vi "Autonomous Independent.vi"   [LabVIEW 2015]
doc: "This VI is called when autonomous begins, and will automatically be terminated when autonomous ends. You can carry out timed or sensor driven robot movement independently without needing to return to the caller."
uses:
  <vilib>/Rock Robotics/WPI/CAN/TalonSRX/WPI_CANTalonSRX_Params.ctl
  <vilib>/Rock Robotics/Network Tables/NT Read Number.vi
  <vilib>/Rock Robotics/Network Tables/NT Read Boolean.vi
  Robot Global Data.vi
  Team900-VIs/navX Library v2/navX Library v2.lvlib
panel:
  # "Be sure to right-click and choose Data Operations>>Make Current Value default if you want to save the array values with the VI"
types:
  T1 = typedef "WPI_MotorControlDeviceRef.ctl" = cluster{"DeviceStatus":errorcluster, "Type":T2, "PWM":cluster{"PWM Channel":T3, "DeadBand":T4}, "CAN":cluster{"Device Number":u8, "Control Mode":T5, "Semaphore":T6, "Max Vout":dbl, "TalonSRX Control Mode":T7}, "Invert":bool}
  T2 = typedef "WPI_MotorControlType.ctl" = enum16{"PWM", "CAN", "CANTalonSRX"}
  T3 = typedef "FPGA_DIOPWMChannel.ctl" = enum8{"PWM 0", "PWM 1", "PWM 2", "PWM 3", "PWM 4", "PWM 5", "PWM 6", "PWM 7", "PWM 8", "PWM 9", "PWM MXP 0", "PWM MXP 1", "PWM MXP 2", "PWM MXP 3", "PWM MXP 4", "PWM MXP 5", "PWM MXP 6", "PWM MXP 7", "PWM MXP 8", "PWM MXP 9", "Invalid"}
  T4 = typedef "WPI_PWMDeadband.ctl" = cluster{"Name":string, "maxPositivePwm":i32, "minPositivePwm":i32, "centerPwm":i32, "maxNegativePwm":i32, "minNegativePwm":i32, "angularRange":u16}
  T5 = typedef "WPI_CANJaguar_ControlMode.ctl" = enum8{"Percent VBus", "Current", "Speed", "Position", "Voltage"}
  T6 = typedef "Semaphore RefNum" = refnum<k1>
  T7 = typedef "WPI_CANTalonSRX_APIControlMode.ctl" = enum8{"Percent VBus", "Speed", "Position", "Slave", "Unchanged / Invalid", "Voltage Compensation", "Current", "Motion Profile"}
  T8 = typedef "WPI_CANTalonSRX_Params.ctl" = u8
  T9 = typedef "navX Library v2.lvlib/Z900_navX_DeviceTypeDef.ctl" = cluster{"Interface":cluster{"Protocol":T10, "Update Rate (4Hz-60Hz)":u8, "navX Open TypeDef":variant}, "Notify Packet":refnum<notifier>, "Loop VI Refnum":refnum<vi>, "Ready to Close Occurrence Refnum":refnum<k4>}
  T10 = typedef "navX Library v2.lvlib/Z900_navX_ProtocolTypeDef.ctl" = enum16{"SERIAL", "I2C", "SPI"}
  T11 = cluster{"Yaw":dbl, "Roll":dbl, "Pitch":dbl, "Heading":dbl, "Fused Heading":dbl}
  T12 = enum16{"nothing", "Fire", "Aim Goal", "Aim Foward"}
  T13 = enum16{"Nothing", "Turn to Angle", "Pick Up Ball", "Drive Straight", "Drive to Target (arc)"}
  T14 = cluster{"X":dbl, "Y":dbl, "Angle":dbl, "Distance":dbl}
  T15 = enum16{"nothing", "intaketotop", "eject ball", "load ball to shooter", "intaketobottom"}
  T16 = typedef "WPI_DigitalInputDevRef.ctl" = cluster{"DevStatus":errorcluster, "DIO Channel":T17}
  T17 = typedef "FPGA_DIOChannel.ctl" = enum8{"DIO 0", "DIO 1", "DIO 2", "DIO 3", "DIO 4", "DIO 5", "DIO 6", "DIO 7", "DIO 8", "DIO 9", "DIO MXP 0", "DIO MXP 1", "DIO MXP 2", "DIO MXP 3", "DIO MXP 4", "DIO MXP 5", "DIO MXP 6", "DIO MXP 7", "DIO MXP 8", "DIO MXP 9", "DIO MXP 10", "DIO MXP 11", "DIO MXP 12", "DIO MXP 13", "DIO MXP 14", "DIO MXP 15", "Invalid"}
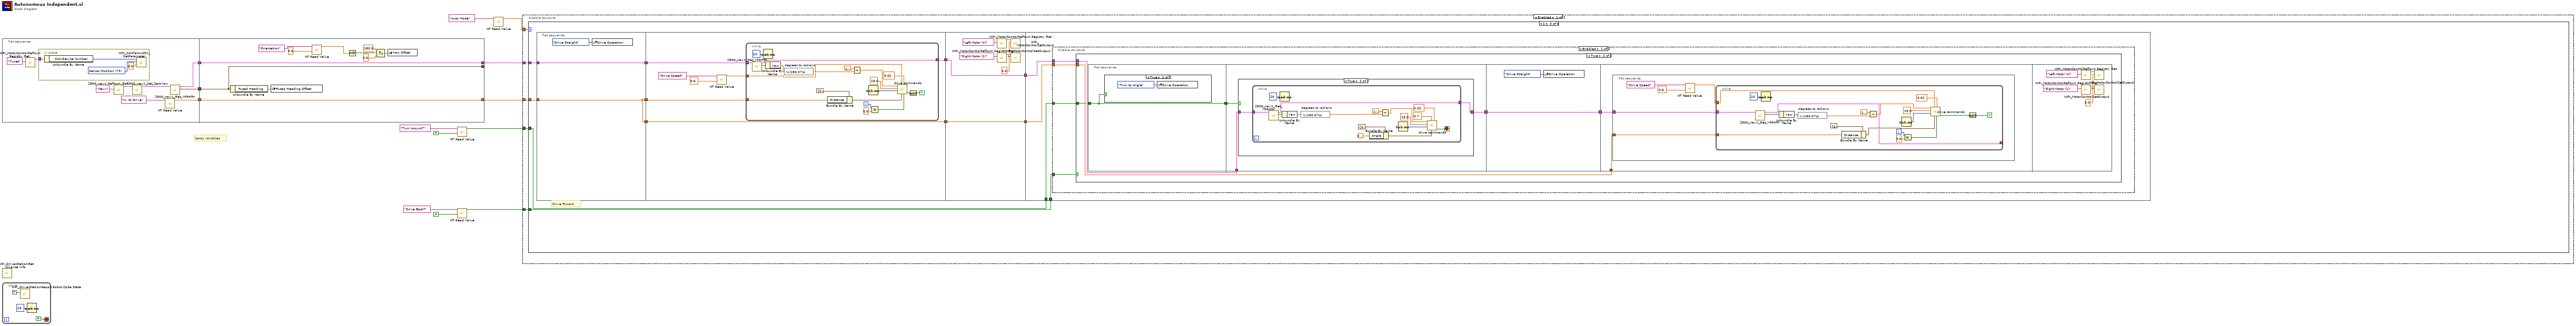
[diagram p0: block diagram]
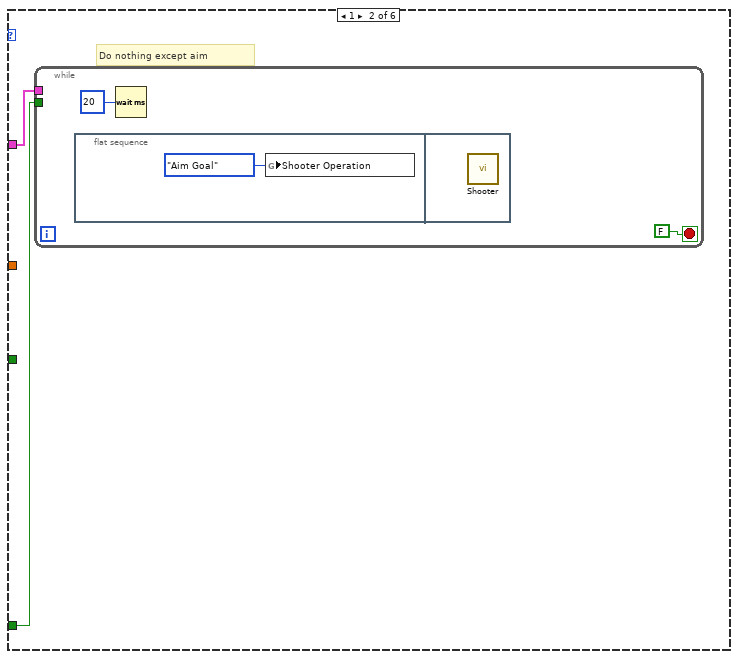
[diagram p3: hidden frame]
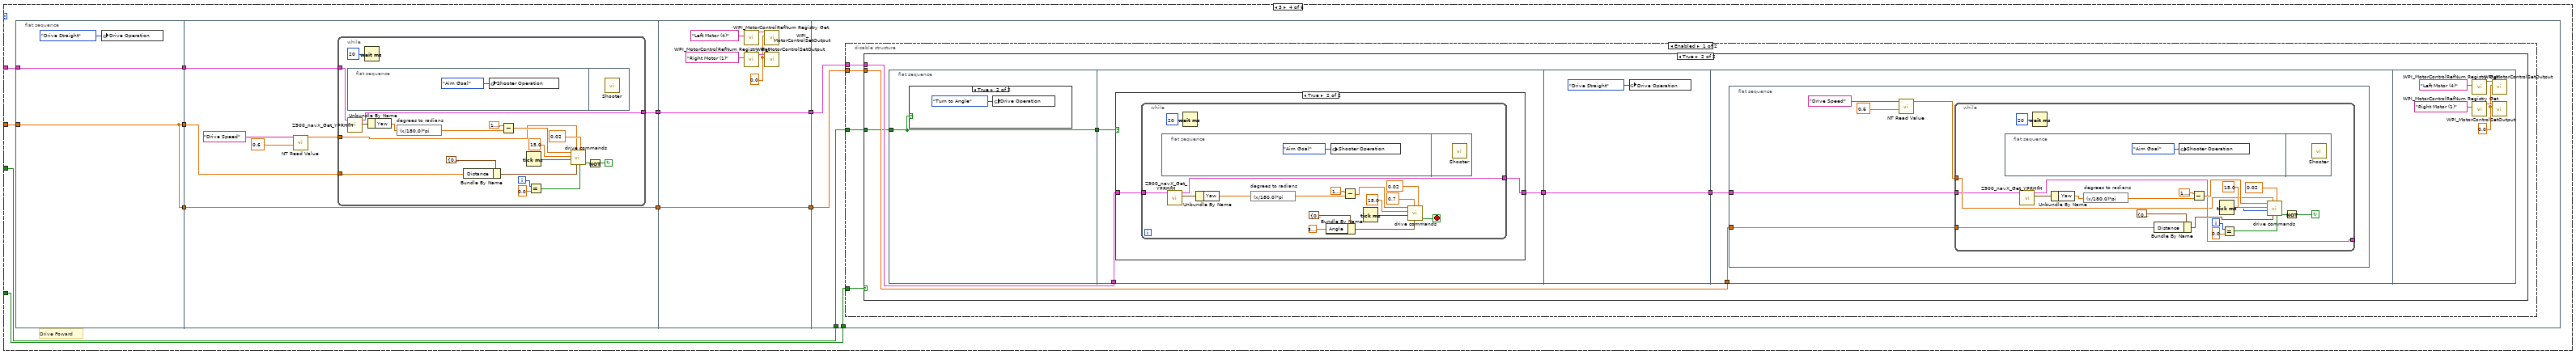
[diagram p8: hidden frame]
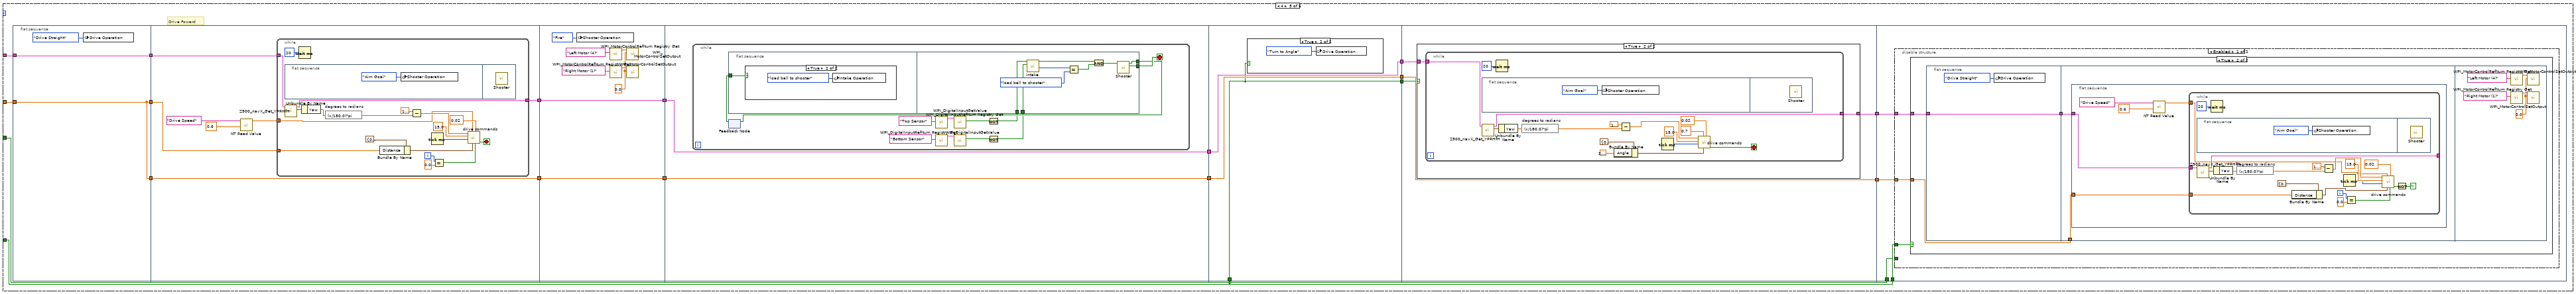
[diagram p13: hidden frame]
diagram:
  # "Zeros variables"
  n1 = flat-sequence {
    tunnel: [w21] -> w3
    tunnel: [w17] -> w2
    tunnel: [w16] -> w1
    tunnel: [w34] -> _
    tunnel: [w36] -> w6
    tunnel: [w37] -> w11
    tunnel: w3 -> [w37]
    tunnel: w2 -> [w36]
    tunnel: w1 -> [w34]
    frame #0 {
      n2 = call <vilib>:"WPI_MotorControlRefNum Registry Get.vi"("refnum name"="Turret") -> ("MotorControlDevRef"=w15:T1)  [unwired: 9 in, 1 out]
      n3 = in-place {
        in-place-border: w15 -> [w26]
        w24 = T8 73 items=["Slot 0 - P"=1, "Slot 0 - I"=2, "Slot 0 - D"=3, "Slot 0 - F"=4, "Slot 0 - I Zone"=5, "Slot 0 - Ramp Rate"=6, "Slot 1 - P"=11, "Slot 1 - I"=12, "Slot 1 - D"=13, "Slot 1 - F"=14, "Slot 1 - I Zone"=15, "Slot 1 - Ramp Rate"=16, "Soft Limit - Forward"=21, "Soft Limit - Reverse"=22, "On Boot - Brake Mode"=31, "On Boot - Limit Normally Closed - Forward"=32, "On Boot - Limit Normally Closed - Reverse"=33, "On Boot - Limit Disabled - Forward"=34, "On Boot - Limit Disabled - Reverse"=35, "Fault - Over Temp"=41, "Fault - Under Voltage"=42, "Fault - Forward Limit"=43, "Fault - Reverse Limit"=44, "Fault - Hardware Failure"=45, "Fault - Forward Soft Limit"=46, "Fault - Reverse Soft Limit"=47, "Sticky Fault - Over Temp"=48, "Sticky Fault - Under Voltage"=49, "Sticky Fault - Forward Limit"=50, "Sticky Fault - Reverse Limit"=51, "Sticky Fault - Forward Soft Limit"=52, "Sticky Fault - Reverse Soft Limit"=53, "Applied Throttle"=61, "Closed-Loop Error"=62, "Select Feedback Device"=63, "Reverse Closed-Loop Output"=64, "Mode Select"=65, "Profile Slot Select"=66, "Ramp Throttle"=67, "Reverse Feedback Sensor"=68, "Limit Switch Enabled"=69, "Limit Switch Closed - Forward"=70, "Limit Switch Closed - Reverse"=71, "Sensor Position"=73, "Sensor Velocity"=74, "Current"=75, "Brake is Enabled"=76, "Encoder Position"=77, "Encoder Velocity"=78, "Encoder Index Rise Events"=79, "Encoder A Pin State"=80, "Encoder B Pin State"=81, "Encoder Index Pin State"=82, "Analog In with Overflow"=83, "Analog In Velocity"=84, "Temperature"=85, "Battery Voltage"=86, "Reset Count"=87, "Reset Flags"=88, "Firmware Version"=89, "Settings Changed"=90] ("Parameter")
        n4 = Unbundle By Name(w26) -> ("CAN.Device Number"=w25:u8)
        n5 = call <vilib>:"WPI_CANTalonSRX_SetParameter.vi"("Value"=0.0, "Parameter"=w24, "Device ID (0)"=w25) -> ()  [unwired: 7 in, 2 out]
      }
      n6 = call "Z900_navX_RefNum_Get.vi"("refnum name"="Navx") -> ("navX Device"=w19:T9)  [unwired: 9 in, 1 out]
      n7 = call "Z900_navX_Set_ZeroYaw.vi"("navX Device"=w19) -> ("navX Device"=w18:T9)  [unwired: 9 in, 1 out]
      n8 = call-poly <vilib>:"NT Read Value.vi"("Name"="In. to Drive") -> ("Numeric"=w21:dbl)  [unwired: 9 in, 1 out]
      n9 = call "Z900_navX_Get_YPRHfH.vi"("navX Device"=w18) -> ("YRPHfH"=w16:T11, "navX Device"=w17:T9)  [unwired: 7 in, 2 out]
    }
    frame #1 {
      n10 = Unbundle By Name(w34) -> ("Fused Heading"=w35:dbl)
      n11 = global write "Robot Global Data.vi" "Fused Heading Offset"(w35) -> ()
      n12 = call-poly <vilib>:"NT Read Value.vi"("Default Value"=0.0, "Name"="Orientation") -> ("Numeric"=w32:dbl)  [unwired: 8 in, 1 out]
      n13 = Equal To 0?(x=w32) -> (x = 0?=w31:bool)
      n14 = Select(t=180.0, s=w31, f=0.0) -> (s? t:f=w28:dbl)
      n15 = global write "Robot Global Data.vi" "Yaw Offset"(w28) -> ()
    }
  }
  n16 = call <vilib>:"WPI_DriverStationGet Alliance Info.vi"() -> ()  [unwired: 12 out]
  n17 = while {
    stop <- FALSE stop-if-true
    n18 = call <vilib>:"WPI_DriverStationReport Robot Code State.vi"("Autonomous"=TRUE) -> ()  [unwired: 10 in, 1 out]
    n19 = Wait (ms)(milliseconds to wait=u32 20) -> ()  [unwired: 1 out]
  }
  n20 = call-poly <vilib>:"NT Read Value.vi"("Default Value"=FALSE, "Name"="Turn Around?") -> ("Boolean"=w7:bool)  [unwired: 8 in, 1 out]
  n21 = call-poly <vilib>:"NT Read Value.vi"("Default Value"=FALSE, "Name"="Drive Back?") -> ("Boolean"=w10:bool)  [unwired: 8 in, 1 out]
  n22 = call-poly <vilib>:"NT Read Value.vi"("Name"="Auto Mode") -> ("Numeric"=w5:dbl)  [unwired: 9 in, 1 out]
  n23 = disable-structure shown="Enabled" {
    disable-tunnel: w5 -> [w45 _]
    disable-tunnel: w6 -> [w44 _]
    disable-tunnel: w11 -> [w43 _]
    disable-tunnel: w10 -> [w42 _]
    disable-tunnel: w7 -> [w41 _]
    frame Enabled {
      n24 = case shown="2" w45 {
        tunnel: w44 -> [_ w47 w61 w181 w311 _]
        tunnel: w43 -> [_ _ w60 w180 w310 _]
        tunnel: w42 -> [_ w46 w57 w177 w307 _]
        tunnel: w41 -> [_ _ w51 w171 w295 _]
        frame 0, Default {
          # "Do nothing"
        }
        frame 1 {
          # "Do nothing except aim"
          n25 = while {
            tunnel: w47 -> [_]
            tunnel: w46 -> [_]
            stop <- FALSE stop-if-true
            n26 = flat-sequence {
              frame #0 {
                n27 = global write "Robot Global Data.vi" "Shooter Operation"(T12."Aim Goal" ("Shooter Operation")) -> ()
              }
              frame #1 {
                n28 = call "Shooter.vi"() -> ()  [unwired: 8 in, 4 out]
              }
            }
            n29 = Wait (ms)(milliseconds to wait=20) -> ()  [unwired: 1 out]
          }
        }
        frame 2 {
          # "Drive Foward"
          n30 = flat-sequence {
            tunnel: w60 -> [w62]
            tunnel: w61 -> [w64]
            tunnel: [w64] -> w59
            tunnel: [w62] -> w58
            tunnel: [w62] -> w54
            tunnel: w59 -> [w71]
            tunnel: w58 -> [w70]
            tunnel: [w69] -> w56
            tunnel: w54 -> [w65]
            tunnel: [w65] -> w53
            tunnel: w56 -> [w98]
            tunnel: [w98] -> w55
            tunnel: w53 -> [w92]
            tunnel: [w92] -> w52
            tunnel: w57 -> [w102]
            tunnel: w55 -> [w101]
            tunnel: w52 -> [w100]
            tunnel: w51 -> [w99]
            frame #0 {
              n31 = global write "Robot Global Data.vi" "Drive Operation"(T13."Drive Straight" ("Drive Operation")) -> ()
            }
            frame #1 {
              n32 = call-poly <vilib>:"NT Read Value.vi"("Default Value"=0.6, "Name"="Drive Speed") -> ("Numeric"=w66:dbl)  [unwired: 8 in, 1 out]
              n33 = while {
                tunnel: w71 -> [w91]
                tunnel: w70 -> [w83]
                tunnel: [w78] -> w69
                tunnel: w66 -> [w72]
                i -> [w75]
                stop <- w76 continue-if-true
                n34 = call "Z900_navX_Get_YPRHfH.vi"("navX Device"=w91) -> ("YRPHfH"=w90:T11, "navX Device"=w78:T9)  [unwired: 7 in, 2 out]
                n35 = Wait (ms)(milliseconds to wait=20) -> ()  [unwired: 1 out]
                n36 = Unbundle By Name(w90) -> ("Yaw"=w87:dbl)
                n37 = expression code="(x/180.0)*pi" "degrees to radians"(w87) -> (w86:dbl)
                n38 = Bundle By Name(cluster=T14 {"X"=0.0, "Y"=0.0, "Angle"=0.0, "Distance"=0.0} ("Position"), "Distance"=w83) -> (w81:T14)
                n39 = Subtract(x=1.5707963267948966, y=w86) -> (x-y=w89:dbl)
                n40 = Tick Count (ms)() -> (millisecond timer value=w84:u32)
                n41 = Equal?(x=w75, y=0.0) -> (x = y?=w73:bool)
                n42 = call "drive commands.vi"("New Command"=w73, "Angle Tolerance"=0.02, "Position"=w81, "Speed Setpoint"=w72, "Current Time"=w84, "Duration"=15.0, "Yaw (radians, 0=right)"=w89) -> ("Finished"=w79:bool)  [unwired: 2 in, 2 out]
                n43 = Not(x=w79) -> (.not. x?=w76:bool)
              }
            }
            frame #2 {
              w93 = 0.0 ("Output")
              n44 = call <vilib>:"WPI_MotorControlRefNum Registry Get.vi"("refnum name"="Left Motor (4)") -> ("MotorControlDevRef"=w94:T1)  [unwired: 9 in, 1 out]
              n45 = call <vilib>:"WPI_MotorControlRefNum Registry Get.vi"("refnum name"="Right Motor (1)") -> ("MotorControlDevRef"=w95:T1)  [unwired: 9 in, 1 out]
              n46 = call <vilib>:"WPI_MotorControlSetOutput.vi"("Output"=w93, "MotorControlDevRef"=w94) -> ()  [unwired: 7 in, 3 out]
              n47 = call <vilib>:"WPI_MotorControlSetOutput.vi"("Output"=w93, "MotorControlDevRef"=w95) -> ()  [unwired: 7 in, 3 out]
            }
            frame #3 {
              n48 = disable-structure shown="Enabled" {
                disable-tunnel: w102 -> [w106 _]
                disable-tunnel: w101 -> [w105 _]
                disable-tunnel: w100 -> [w104 _]
                disable-tunnel: w99 -> [w103 _]
                frame Enabled {
                  n49 = case shown="True" w106 {
                    tunnel: w105 -> [_ w112]
                    tunnel: w104 -> [_ w110]
                    tunnel: w103 -> [_ w109]
                    frame False {
                    }
                    frame True {
                      n50 = flat-sequence {
                        tunnel: w109 -> [w113]
                        tunnel: [w113] -> w108
                        tunnel: w112 -> [w117]
                        tunnel: [w116] -> w111
                        tunnel: w108 -> [w115]
                        tunnel: w111 -> [w137]
                        tunnel: [w137] -> w107
                        tunnel: w110 -> [w140]
                        tunnel: w107 -> [w139]
                        frame #0 {
                          n51 = case shown="True" w113 {
                            frame False {
                            }
                            frame True {
                              n52 = global write "Robot Global Data.vi" "Drive Operation"(T13."Turn to Angle" ("Drive Operation")) -> ()
                            }
                          }
                        }
                        frame #1 {
                          n53 = case shown="True" w115 {
                            tunnel: w117 -> [w118 w120]
                            tunnel: [w118 w119] -> w116
                            frame False {
                            }
                            frame True {
                              n54 = while {
                                tunnel: w120 -> [w136]
                                tunnel: [w121] -> w119
                                stop <- w124 stop-if-true
                                n55 = call "Z900_navX_Get_YPRHfH.vi"("navX Device"=w136) -> ("YRPHfH"=w135:T11, "navX Device"=w121:T9)  [unwired: 7 in, 2 out]
                                n56 = Wait (ms)(milliseconds to wait=20) -> ()  [unwired: 1 out]
                                n57 = Unbundle By Name(w135) -> ("Yaw"=w132:dbl)
                                n58 = expression code="(x/180.0)*pi" "degrees to radians"(w132) -> (w131:dbl)
                                n59 = Bundle By Name(cluster=T14 {"X"=0.0, "Y"=0.0, "Angle"=0.0, "Distance"=0.0} ("Position"), "Angle"=3.141592653589793) -> (w127:T14)
                                n60 = Subtract(x=1.5707963267948966, y=w131) -> (x-y=w134:dbl)
                                n61 = Tick Count (ms)() -> (millisecond timer value=w129:u32)
                                n62 = call "drive commands.vi"("Angle Tolerance"=0.02, "Position"=w127, "Speed Setpoint"=0.7, "Current Time"=w129, "Duration"=15.0, "Yaw (radians, 0=right)"=w134) -> ("Finished"=w124:bool)  [unwired: 3 in, 2 out]
                              }
                            }
                          }
                        }
                        frame #2 {
                          n63 = global write "Robot Global Data.vi" "Drive Operation"(T13."Drive Straight" ("Drive Operation")) -> ()
                        }
                        frame #3 {
                          n64 = flat-sequence {
                            tunnel: w140 -> [w142]
                            tunnel: w139 -> [w141]
                            frame #0 {
                              n65 = call-poly <vilib>:"NT Read Value.vi"("Default Value"=0.6, "Name"="Drive Speed") -> ("Numeric"=w143:dbl)  [unwired: 8 in, 1 out]
                              n66 = while {
                                tunnel: [w154] -> _
                                tunnel: w143 -> [w148]
                                tunnel: w142 -> [w147]
                                tunnel: w141 -> [w146]
                                i -> [w151]
                                stop <- w152 continue-if-true
                                n67 = call "Z900_navX_Get_YPRHfH.vi"("navX Device"=w146) -> ("YRPHfH"=w165:T11, "navX Device"=w154:T9)  [unwired: 7 in, 2 out]
                                n68 = Wait (ms)(milliseconds to wait=20) -> ()  [unwired: 1 out]
                                n69 = Unbundle By Name(w165) -> ("Yaw"=w162:dbl)
                                n70 = expression code="(x/180.0)*pi" "degrees to radians"(w162) -> (w161:dbl)
                                n71 = Bundle By Name(cluster=T14 {"X"=0.0, "Y"=0.0, "Angle"=0.0, "Distance"=0.0} ("Position"), "Distance"=w147) -> (w157:T14)
                                n72 = Subtract(x=1.5707963267948966, y=w161) -> (x-y=w164:dbl)
                                n73 = Tick Count (ms)() -> (millisecond timer value=w159:u32)
                                n74 = Equal?(x=w151, y=0.0) -> (x = y?=w149:bool)
                                n75 = call "drive commands.vi"("New Command"=w149, "Angle Tolerance"=0.02, "Position"=w157, "Speed Setpoint"=w148, "Current Time"=w159, "Duration"=15.0, "Yaw (radians, 0=right)"=w164) -> ("Finished"=w155:bool)  [unwired: 2 in, 2 out]
                                n76 = Not(x=w155) -> (.not. x?=w152:bool)
                              }
                            }
                          }
                        }
                        frame #4 {
                          w166 = 0.0 ("Output")
                          n77 = call <vilib>:"WPI_MotorControlRefNum Registry Get.vi"("refnum name"="Left Motor (4)") -> ("MotorControlDevRef"=w167:T1)  [unwired: 9 in, 1 out]
                          n78 = call <vilib>:"WPI_MotorControlRefNum Registry Get.vi"("refnum name"="Right Motor (1)") -> ("MotorControlDevRef"=w168:T1)  [unwired: 9 in, 1 out]
                          n79 = call <vilib>:"WPI_MotorControlSetOutput.vi"("Output"=w166, "MotorControlDevRef"=w167) -> ()  [unwired: 7 in, 3 out]
                          n80 = call <vilib>:"WPI_MotorControlSetOutput.vi"("Output"=w166, "MotorControlDevRef"=w168) -> ()  [unwired: 7 in, 3 out]
                        }
                      }
                    }
                  }
                }
                frame Disabled {
                }
              }
            }
          }
        }
        frame 3 {
          # "Drive Foward"
          n81 = flat-sequence {
            tunnel: w180 -> [w182]
            tunnel: w181 -> [w184]
            tunnel: [w184] -> w179
            tunnel: [w182] -> w178
            tunnel: [w182] -> w174
            tunnel: w179 -> [w191]
            tunnel: w178 -> [w190]
            tunnel: [w189] -> w176
            tunnel: w174 -> [w185]
            tunnel: [w185] -> w173
            tunnel: w176 -> [w219]
            tunnel: [w219] -> w175
            tunnel: w173 -> [w213]
            tunnel: [w213] -> w172
            tunnel: w177 -> [w223]
            tunnel: w175 -> [w222]
            tunnel: w172 -> [w221]
            tunnel: w171 -> [w220]
            frame #0 {
              n82 = global write "Robot Global Data.vi" "Drive Operation"(T13."Drive Straight" ("Drive Operation")) -> ()
            }
            frame #1 {
              n83 = call-poly <vilib>:"NT Read Value.vi"("Default Value"=0.6, "Name"="Drive Speed") -> ("Numeric"=w186:dbl)  [unwired: 8 in, 1 out]
              n84 = while {
                tunnel: w191 -> [w211]
                tunnel: w190 -> [w203]
                tunnel: [w198] -> w189
                tunnel: w186 -> [w192]
                i -> [w195]
                stop <- w196 continue-if-true
                n85 = flat-sequence {
                  frame #0 {
                    n86 = global write "Robot Global Data.vi" "Shooter Operation"(T12."Aim Goal" ("Shooter Operation")) -> ()
                  }
                  frame #1 {
                    n87 = call "Shooter.vi"() -> ()  [unwired: 8 in, 4 out]
                  }
                }
                n88 = call "Z900_navX_Get_YPRHfH.vi"("navX Device"=w211) -> ("YRPHfH"=w210:T11, "navX Device"=w198:T9)  [unwired: 7 in, 2 out]
                n89 = Wait (ms)(milliseconds to wait=20) -> ()  [unwired: 1 out]
                n90 = Unbundle By Name(w210) -> ("Yaw"=w207:dbl)
                n91 = expression code="(x/180.0)*pi" "degrees to radians"(w207) -> (w206:dbl)
                n92 = Bundle By Name(cluster=T14 {"X"=0.0, "Y"=0.0, "Angle"=0.0, "Distance"=0.0} ("Position"), "Distance"=w203) -> (w201:T14)
                n93 = Subtract(x=1.5707963267948966, y=w206) -> (x-y=w209:dbl)
                n94 = Tick Count (ms)() -> (millisecond timer value=w204:u32)
                n95 = Equal?(x=w195, y=0.0) -> (x = y?=w193:bool)
                n96 = call "drive commands.vi"("New Command"=w193, "Angle Tolerance"=0.02, "Position"=w201, "Speed Setpoint"=w192, "Current Time"=w204, "Duration"=15.0, "Yaw (radians, 0=right)"=w209) -> ("Finished"=w199:bool)  [unwired: 2 in, 2 out]
                n97 = Not(x=w199) -> (.not. x?=w196:bool)
              }
            }
            frame #2 {
              w214 = 0.0 ("Output")
              n98 = call <vilib>:"WPI_MotorControlRefNum Registry Get.vi"("refnum name"="Left Motor (4)") -> ("MotorControlDevRef"=w215:T1)  [unwired: 9 in, 1 out]
              n99 = call <vilib>:"WPI_MotorControlRefNum Registry Get.vi"("refnum name"="Right Motor (1)") -> ("MotorControlDevRef"=w216:T1)  [unwired: 9 in, 1 out]
              n100 = call <vilib>:"WPI_MotorControlSetOutput.vi"("Output"=w214, "MotorControlDevRef"=w215) -> ()  [unwired: 7 in, 3 out]
              n101 = call <vilib>:"WPI_MotorControlSetOutput.vi"("Output"=w214, "MotorControlDevRef"=w216) -> ()  [unwired: 7 in, 3 out]
            }
            frame #3 {
              n102 = disable-structure shown="Enabled" {
                disable-tunnel: w223 -> [w227 _]
                disable-tunnel: w222 -> [w226 _]
                disable-tunnel: w221 -> [w225 _]
                disable-tunnel: w220 -> [w224 _]
                frame Enabled {
                  n103 = case shown="True" w227 {
                    tunnel: w226 -> [_ w233]
                    tunnel: w225 -> [_ w231]
                    tunnel: w224 -> [_ w230]
                    frame False {
                    }
                    frame True {
                      n104 = flat-sequence {
                        tunnel: w230 -> [w234]
                        tunnel: [w234] -> w229
                        tunnel: w233 -> [w238]
                        tunnel: [w237] -> w232
                        tunnel: w229 -> [w236]
                        tunnel: w232 -> [w259]
                        tunnel: [w259] -> w228
                        tunnel: w231 -> [w262]
                        tunnel: w228 -> [w261]
                        frame #0 {
                          n105 = case shown="True" w234 {
                            frame False {
                            }
                            frame True {
                              n106 = global write "Robot Global Data.vi" "Drive Operation"(T13."Turn to Angle" ("Drive Operation")) -> ()
                            }
                          }
                        }
                        frame #1 {
                          n107 = case shown="True" w236 {
                            tunnel: w238 -> [w239 w241]
                            tunnel: [w239 w240] -> w237
                            frame False {
                            }
                            frame True {
                              n108 = while {
                                tunnel: w241 -> [w257]
                                tunnel: [w242] -> w240
                                stop <- w245 stop-if-true
                                n109 = flat-sequence {
                                frame #0 {
                                n110 = global write "Robot Global Data.vi" "Shooter Operation"(T12."Aim Goal" ("Shooter Operation")) -> ()
                                }
                                frame #1 {
                                n111 = call "Shooter.vi"() -> ()  [unwired: 8 in, 4 out]
                                }
                                }
                                n112 = call "Z900_navX_Get_YPRHfH.vi"("navX Device"=w257) -> ("YRPHfH"=w256:T11, "navX Device"=w242:T9)  [unwired: 7 in, 2 out]
                                n113 = Wait (ms)(milliseconds to wait=20) -> ()  [unwired: 1 out]
                                n114 = Unbundle By Name(w256) -> ("Yaw"=w253:dbl)
                                n115 = expression code="(x/180.0)*pi" "degrees to radians"(w253) -> (w252:dbl)
                                n116 = Bundle By Name(cluster=T14 {"X"=0.0, "Y"=0.0, "Angle"=0.0, "Distance"=0.0} ("Position"), "Angle"=3.141592653589793) -> (w248:T14)
                                n117 = Subtract(x=1.5707963267948966, y=w252) -> (x-y=w255:dbl)
                                n118 = Tick Count (ms)() -> (millisecond timer value=w250:u32)
                                n119 = call "drive commands.vi"("Angle Tolerance"=0.02, "Position"=w248, "Speed Setpoint"=0.7, "Current Time"=w250, "Duration"=15.0, "Yaw (radians, 0=right)"=w255) -> ("Finished"=w245:bool)  [unwired: 3 in, 2 out]
                              }
                            }
                          }
                        }
                        frame #2 {
                          n120 = global write "Robot Global Data.vi" "Drive Operation"(T13."Drive Straight" ("Drive Operation")) -> ()
                        }
                        frame #3 {
                          n121 = flat-sequence {
                            tunnel: w262 -> [w264]
                            tunnel: w261 -> [w263]
                            frame #0 {
                              n122 = call-poly <vilib>:"NT Read Value.vi"("Default Value"=0.6, "Name"="Drive Speed") -> ("Numeric"=w265:dbl)  [unwired: 8 in, 1 out]
                              n123 = while {
                                tunnel: [w276] -> _
                                tunnel: w265 -> [w270]
                                tunnel: w264 -> [w269]
                                tunnel: w263 -> [w268]
                                i -> [w273]
                                stop <- w274 continue-if-true
                                n124 = flat-sequence {
                                frame #0 {
                                n125 = global write "Robot Global Data.vi" "Shooter Operation"(T12."Aim Goal" ("Shooter Operation")) -> ()
                                }
                                frame #1 {
                                n126 = call "Shooter.vi"() -> ()  [unwired: 8 in, 4 out]
                                }
                                }
                                n127 = call "Z900_navX_Get_YPRHfH.vi"("navX Device"=w268) -> ("YRPHfH"=w287:T11, "navX Device"=w276:T9)  [unwired: 7 in, 2 out]
                                n128 = Wait (ms)(milliseconds to wait=20) -> ()  [unwired: 1 out]
                                n129 = Unbundle By Name(w287) -> ("Yaw"=w284:dbl)
                                n130 = expression code="(x/180.0)*pi" "degrees to radians"(w284) -> (w283:dbl)
                                n131 = Bundle By Name(cluster=T14 {"X"=0.0, "Y"=0.0, "Angle"=0.0, "Distance"=0.0} ("Position"), "Distance"=w269) -> (w279:T14)
                                n132 = Subtract(x=1.5707963267948966, y=w283) -> (x-y=w286:dbl)
                                n133 = Tick Count (ms)() -> (millisecond timer value=w281:u32)
                                n134 = Equal?(x=w273, y=0.0) -> (x = y?=w271:bool)
                                n135 = call "drive commands.vi"("New Command"=w271, "Angle Tolerance"=0.02, "Position"=w279, "Speed Setpoint"=w270, "Current Time"=w281, "Duration"=15.0, "Yaw (radians, 0=right)"=w286) -> ("Finished"=w277:bool)  [unwired: 2 in, 2 out]
                                n136 = Not(x=w277) -> (.not. x?=w274:bool)
                              }
                            }
                          }
                        }
                        frame #4 {
                          w289 = 0.0 ("Output")
                          n137 = call <vilib>:"WPI_MotorControlRefNum Registry Get.vi"("refnum name"="Left Motor (4)") -> ("MotorControlDevRef"=w290:T1)  [unwired: 9 in, 1 out]
                          n138 = call <vilib>:"WPI_MotorControlRefNum Registry Get.vi"("refnum name"="Right Motor (1)") -> ("MotorControlDevRef"=w291:T1)  [unwired: 9 in, 1 out]
                          n139 = call <vilib>:"WPI_MotorControlSetOutput.vi"("Output"=w289, "MotorControlDevRef"=w290) -> ()  [unwired: 7 in, 3 out]
                          n140 = call <vilib>:"WPI_MotorControlSetOutput.vi"("Output"=w289, "MotorControlDevRef"=w291) -> ()  [unwired: 7 in, 3 out]
                        }
                      }
                    }
                  }
                }
                frame Disabled {
                }
              }
            }
          }
        }
        frame 4 {
          # "Drive Foward"
          n141 = flat-sequence {
            tunnel: w310 -> [w312]
            tunnel: w311 -> [w314]
            tunnel: [w314] -> w309
            tunnel: [w312] -> w308
            tunnel: [w312] -> w305
            tunnel: w309 -> [w321]
            tunnel: w308 -> [w320]
            tunnel: [w319] -> w306
            tunnel: w305 -> [w315]
            tunnel: [w315] -> w304
            tunnel: w306 -> [w349]
            tunnel: [w349] -> w303
            tunnel: w304 -> [w343]
            tunnel: [w343] -> w302
            tunnel: w303 -> [w351]
            tunnel: [w351] -> w301
            tunnel: w302 -> [w350]
            tunnel: [w350] -> w300
            tunnel: w301 -> [w376]
            tunnel: [w376] -> w299
            tunnel: w300 -> [w375]
            tunnel: [w375] -> w297
            tunnel: w295 -> [w374]
            tunnel: [w374] -> w294
            tunnel: w299 -> [w380]
            tunnel: [w379] -> w298
            tunnel: w297 -> [w381]
            tunnel: [w381] -> w296
            tunnel: w294 -> [w378]
            tunnel: w307 -> [w405]
            tunnel: w298 -> [w404]
            tunnel: w296 -> [w403]
            tunnel: w295 -> [w402]
            frame #0 {
              n142 = global write "Robot Global Data.vi" "Drive Operation"(T13."Drive Straight" ("Drive Operation")) -> ()
            }
            frame #1 {
              n143 = call-poly <vilib>:"NT Read Value.vi"("Default Value"=0.6, "Name"="Drive Speed") -> ("Numeric"=w316:dbl)  [unwired: 8 in, 1 out]
              n144 = while {
                tunnel: w321 -> [w340]
                tunnel: w320 -> [w332]
                tunnel: [w328] -> w319
                tunnel: w316 -> [w323]
                i -> [w326]
                stop <- w322 stop-if-true
                n145 = flat-sequence {
                  frame #0 {
                    n146 = global write "Robot Global Data.vi" "Shooter Operation"(T12."Aim Goal" ("Shooter Operation")) -> ()
                  }
                  frame #1 {
                    n147 = call "Shooter.vi"() -> ()  [unwired: 8 in, 4 out]
                  }
                }
                n148 = call "Z900_navX_Get_YPRHfH.vi"("navX Device"=w340) -> ("YRPHfH"=w339:T11, "navX Device"=w328:T9)  [unwired: 7 in, 2 out]
                n149 = Wait (ms)(milliseconds to wait=20) -> ()  [unwired: 1 out]
                n150 = Unbundle By Name(w339) -> ("Yaw"=w336:dbl)
                n151 = expression code="(x/180.0)*pi" "degrees to radians"(w336) -> (w335:dbl)
                n152 = Bundle By Name(cluster=T14 {"X"=0.0, "Y"=0.0, "Angle"=0.0, "Distance"=0.0} ("Position"), "Distance"=w332) -> (w330:T14)
                n153 = Subtract(x=1.5707963267948966, y=w335) -> (x-y=w338:dbl)
                n154 = Tick Count (ms)() -> (millisecond timer value=w333:u32)
                n155 = Equal?(x=w326, y=0.0) -> (x = y?=w324:bool)
                n156 = call "drive commands.vi"("New Command"=w324, "Angle Tolerance"=0.02, "Position"=w330, "Speed Setpoint"=w323, "Current Time"=w333, "Duration"=15.0, "Yaw (radians, 0=right)"=w338) -> ("Finished"=w322:bool)  [unwired: 2 in, 2 out]
              }
            }
            frame #2 {
              w344 = 0.0 ("Output")
              n157 = global write "Robot Global Data.vi" "Shooter Operation"(T12."Fire" ("Shooter Operation")) -> ()
              n158 = call <vilib>:"WPI_MotorControlRefNum Registry Get.vi"("refnum name"="Left Motor (4)") -> ("MotorControlDevRef"=w345:T1)  [unwired: 9 in, 1 out]
              n159 = call <vilib>:"WPI_MotorControlRefNum Registry Get.vi"("refnum name"="Right Motor (1)") -> ("MotorControlDevRef"=w346:T1)  [unwired: 9 in, 1 out]
              n160 = call <vilib>:"WPI_MotorControlSetOutput.vi"("Output"=w344, "MotorControlDevRef"=w345) -> ()  [unwired: 7 in, 3 out]
              n161 = call <vilib>:"WPI_MotorControlSetOutput.vi"("Output"=w344, "MotorControlDevRef"=w346) -> ()  [unwired: 7 in, 3 out]
            }
            frame #3 {
              n162 = while {
                stop <- w362 stop-if-true
                n163 = flat-sequence {
                  tunnel: w360 -> [w363]
                  tunnel: [w373] -> w362
                  tunnel: [w367] -> w361
                  tunnel: w353 -> [w366]
                  tunnel: w352 -> [w365]
                  frame #0 {
                    n164 = case shown="True" w363 {
                      frame False {
                      }
                      frame True {
                        n165 = global write "Robot Global Data.vi" "Intake Operation"(T15."load ball to shooter" ("Intake Operation")) -> ()
                      }
                    }
                  }
                  frame #1 {
                    n166 = call "intake.vi"("Bottom Sensor"=w365, "Top Sensor"=w366) -> ("Intake Operation"=w369:T15, "Operation finished"=w372:bool)  [unwired: 6 in, 2 out]
                    n167 = Equal?(x=w369, y=T15."load ball to shooter") -> (x = y?=w371:bool)
                    n168 = And(x=w372, y=w371) -> (x .and. y?=w370:bool)
                    n169 = call "Shooter.vi"("Load Ball Finished"=w370) -> ("Finished"=w373:bool, "Load Ball"=w367:bool)  [unwired: 7 in, 2 out]
                  }
                }
                n170 = feedback-in #1(w361) -> ()
                n171 = feedback #1() -> (w360:bool)  [unwired: 1 in]
                n172 = call <vilib>:"WPI_DigitalInputRefNum Registry Get.vi"("refnum name"="Top Sensor") -> ("DigitalInputDevRef"=w359:T16)  [unwired: 9 in, 1 out]
                n173 = call <vilib>:"WPI_DigitalInputRefNum Registry Get.vi"("refnum name"="Bottom Sensor") -> ("DigitalInputDevRef"=w356:T16)  [unwired: 9 in, 1 out]
                n174 = call <vilib>:"WPI_DigitalInputGetValue.vi"("DigitalInputDevRef"=w359) -> ("Value"=w358:bool)  [unwired: 8 in, 2 out]
                n175 = call <vilib>:"WPI_DigitalInputGetValue.vi"("DigitalInputDevRef"=w356) -> ("Value"=w355:bool)  [unwired: 8 in, 2 out]
                n176 = Not(x=w358) -> (.not. x?=w353:bool)
                n177 = Not(x=w355) -> (.not. x?=w352:bool)
              }
            }
            frame #4 {
              n178 = case shown="True" w374 {
                frame False {
                }
                frame True {
                  n179 = global write "Robot Global Data.vi" "Drive Operation"(T13."Turn to Angle" ("Drive Operation")) -> ()
                }
              }
            }
            frame #5 {
              n180 = case shown="True" w378 {
                tunnel: w380 -> [w382 w384]
                tunnel: [w382 w383] -> w379
                frame False {
                }
                frame True {
                  n181 = while {
                    tunnel: w384 -> [w400]
                    tunnel: [w385] -> w383
                    stop <- w388 stop-if-true
                    n182 = flat-sequence {
                      frame #0 {
                        n183 = global write "Robot Global Data.vi" "Shooter Operation"(T12."Aim Goal" ("Shooter Operation")) -> ()
                      }
                      frame #1 {
                        n184 = call "Shooter.vi"() -> ()  [unwired: 8 in, 4 out]
                      }
                    }
                    n185 = call "Z900_navX_Get_YPRHfH.vi"("navX Device"=w400) -> ("YRPHfH"=w399:T11, "navX Device"=w385:T9)  [unwired: 7 in, 2 out]
                    n186 = Wait (ms)(milliseconds to wait=20) -> ()  [unwired: 1 out]
                    n187 = Unbundle By Name(w399) -> ("Yaw"=w396:dbl)
                    n188 = expression code="(x/180.0)*pi" "degrees to radians"(w396) -> (w395:dbl)
                    n189 = Bundle By Name(cluster=T14 {"X"=0.0, "Y"=0.0, "Angle"=0.0, "Distance"=0.0} ("Position"), "Angle"=3.141592653589793) -> (w391:T14)
                    n190 = Subtract(x=1.5707963267948966, y=w395) -> (x-y=w398:dbl)
                    n191 = Tick Count (ms)() -> (millisecond timer value=w393:u32)
                    n192 = call "drive commands.vi"("Angle Tolerance"=0.02, "Position"=w391, "Speed Setpoint"=0.7, "Current Time"=w393, "Duration"=15.0, "Yaw (radians, 0=right)"=w398) -> ("Finished"=w388:bool)  [unwired: 3 in, 2 out]
                  }
                }
              }
            }
            frame #6 {
              n193 = disable-structure shown="Enabled" {
                disable-tunnel: w405 -> [w408 _]
                disable-tunnel: w404 -> [w407 _]
                disable-tunnel: w403 -> [w406 _]
                disable-tunnel: w402 -> [_ _]
                frame Enabled {
                  n194 = case shown="True" w408 {
                    tunnel: w407 -> [_ w409]
                    tunnel: w406 -> [_ w411]
                    frame False {
                    }
                    frame True {
                      n195 = flat-sequence {
                        tunnel: [w412] -> w410
                        tunnel: w409 -> [w412]
                        tunnel: w411 -> [w415]
                        tunnel: w410 -> [w414]
                        frame #0 {
                          n196 = global write "Robot Global Data.vi" "Drive Operation"(T13."Drive Straight" ("Drive Operation")) -> ()
                        }
                        frame #1 {
                          n197 = flat-sequence {
                            tunnel: w415 -> [w417]
                            tunnel: w414 -> [w416]
                            frame #0 {
                              n198 = call-poly <vilib>:"NT Read Value.vi"("Default Value"=0.6, "Name"="Drive Speed") -> ("Numeric"=w418:dbl)  [unwired: 8 in, 1 out]
                              n199 = while {
                                tunnel: [w429] -> _
                                tunnel: w418 -> [w423]
                                tunnel: w417 -> [w422]
                                tunnel: w416 -> [w421]
                                i -> [w426]
                                stop <- w427 continue-if-true
                                n200 = flat-sequence {
                                frame #0 {
                                n201 = global write "Robot Global Data.vi" "Shooter Operation"(T12."Aim Goal" ("Shooter Operation")) -> ()
                                }
                                frame #1 {
                                n202 = call "Shooter.vi"() -> ()  [unwired: 8 in, 4 out]
                                }
                                }
                                n203 = call "Z900_navX_Get_YPRHfH.vi"("navX Device"=w421) -> ("YRPHfH"=w440:T11, "navX Device"=w429:T9)  [unwired: 7 in, 2 out]
                                n204 = Wait (ms)(milliseconds to wait=20) -> ()  [unwired: 1 out]
                                n205 = Unbundle By Name(w440) -> ("Yaw"=w437:dbl)
                                n206 = expression code="(x/180.0)*pi" "degrees to radians"(w437) -> (w436:dbl)
                                n207 = Bundle By Name(cluster=T14 {"X"=0.0, "Y"=0.0, "Angle"=0.0, "Distance"=0.0} ("Position"), "Distance"=w422) -> (w432:T14)
                                n208 = Subtract(x=1.5707963267948966, y=w436) -> (x-y=w439:dbl)
                                n209 = Tick Count (ms)() -> (millisecond timer value=w434:u32)
                                n210 = Equal?(x=w426, y=0.0) -> (x = y?=w424:bool)
                                n211 = call "drive commands.vi"("New Command"=w424, "Angle Tolerance"=0.02, "Position"=w432, "Speed Setpoint"=w423, "Current Time"=w434, "Duration"=15.0, "Yaw (radians, 0=right)"=w439) -> ("Finished"=w430:bool)  [unwired: 2 in, 2 out]
                                n212 = Not(x=w430) -> (.not. x?=w427:bool)
                              }
                            }
                          }
                        }
                        frame #2 {
                          w442 = 0.0 ("Output")
                          n213 = call <vilib>:"WPI_MotorControlRefNum Registry Get.vi"("refnum name"="Left Motor (4)") -> ("MotorControlDevRef"=w443:T1)  [unwired: 9 in, 1 out]
                          n214 = call <vilib>:"WPI_MotorControlRefNum Registry Get.vi"("refnum name"="Right Motor (1)") -> ("MotorControlDevRef"=w444:T1)  [unwired: 9 in, 1 out]
                          n215 = call <vilib>:"WPI_MotorControlSetOutput.vi"("Output"=w442, "MotorControlDevRef"=w443) -> ()  [unwired: 7 in, 3 out]
                          n216 = call <vilib>:"WPI_MotorControlSetOutput.vi"("Output"=w442, "MotorControlDevRef"=w444) -> ()  [unwired: 7 in, 3 out]
                        }
                      }
                    }
                  }
                }
                frame Disabled {
                }
              }
            }
          }
        }
        frame 5 {
        }
      }
    }
    frame Disabled {
    }
  }
